vi "SUB_FindSpecificString_After.vi"(3 "Find this String":string, 4 "Before this end token":string, 5 "String data":string) -> (0 "before \"; \" string":string, 1 "after substring":string, 2 "Found":bool)   [LabVIEW 2011]
panel:
  out "match substring":string
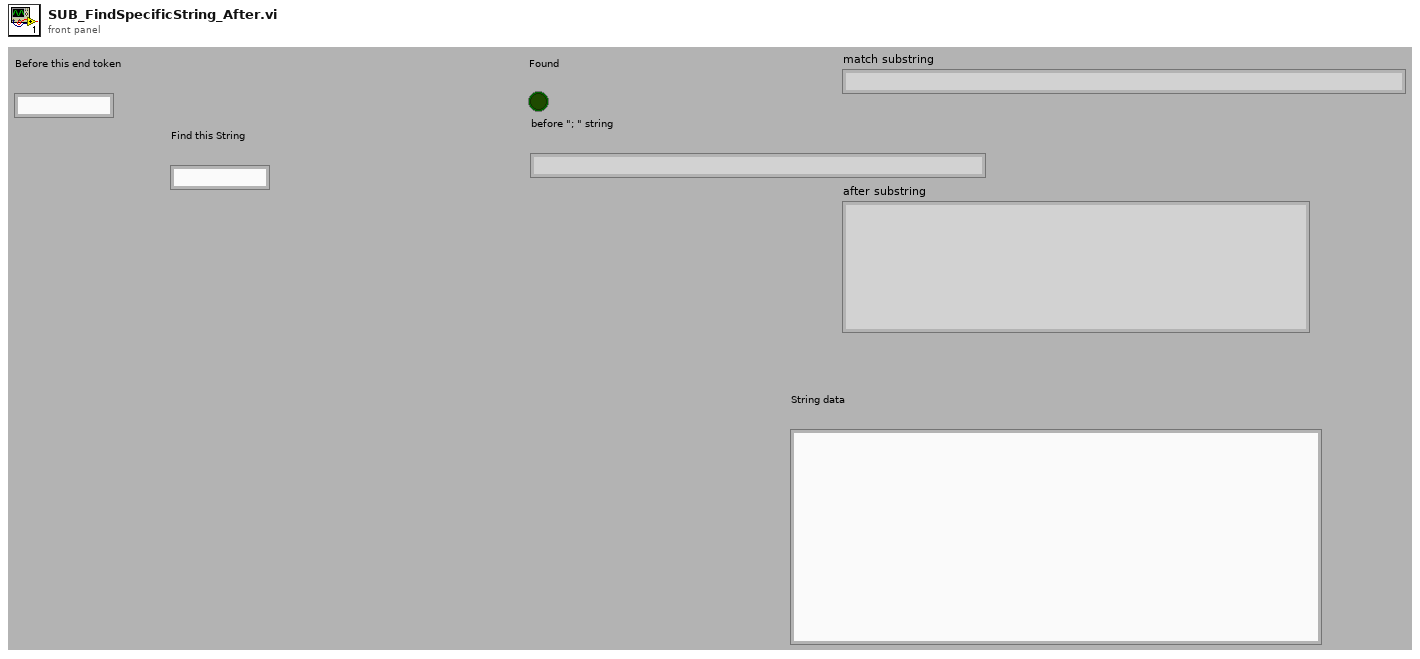
[diagram p1: front panel]
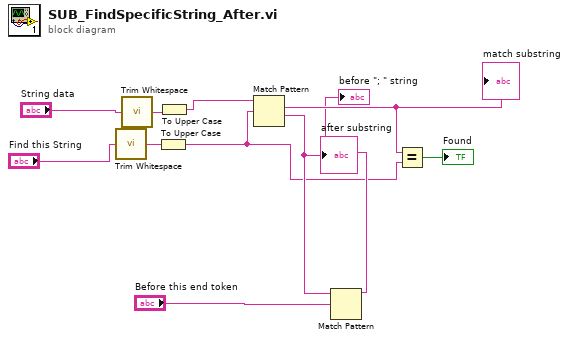
[diagram p0: block diagram]
diagram:
  n1 = call <vilib>:"Trim Whitespace.vi"("string"="Find this String") -> ("trimmed string"=w3:string)  [unwired: 1 in]
  n2 = call <vilib>:"Trim Whitespace.vi"("string"="String data") -> ("trimmed string"=w5:string)  [unwired: 1 in]
  n3 = To Upper Case(1:w3) -> (0:w2:string)
  n4 = To Upper Case(1:w5) -> (0:w4:string)
  n5 = Match Pattern(string=w4, regular expression=w2) -> (match substring=w10:string, after substring=w11:string)  [unwired: 1 in, 2 out]
  "match substring" <- w10
  "after substring" <- w11
  n6 = Match Pattern(string=w11, regular expression="Before this end token") -> (before substring=→"before \"; \" string":string)  [unwired: 1 in, 3 out]
  n7 = Equal?(x=w10, y=w2) -> (x = y?=→"Found":bool)
